vi "GetCursor.vi"(1 "Active Cursor":u32, 2 "WFGraph Refnum":refnum<vi>) -> (0 "Cursor.Cursor X":dbl)   [LabVIEW 2009]
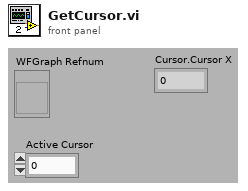
[diagram p1: front panel]
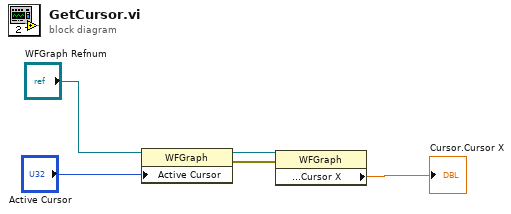
[diagram p0: block diagram]
diagram:
  n1 = property class="WFGraph"(reference="WFGraph Refnum", "Active Cursor"="Active Cursor") -> (reference out=w2:refnum<vi>, error out=w1:errorcluster)  [unwired: 1 in]
  n2 = property class="WFGraph"(reference=w2, error in=w1) -> ("Cursor.Cursor Position:Cursor X"=→"Cursor.Cursor X":dbl)  [unwired: 2 out]
